vi "Trim end of multiline string of CRLFs and just have one CRLF.vi"(8 "error in (no error)":errorcluster, 11 "String in":string) -> (0 "error out":errorcluster, 1 "Delimiter":string, 2 "String out":string, 3 "Line cnt":i32)   [LabVIEW 2013]
doc: "Removes end of multiline string whitespace on just the last line and puts one lf there so string is just the number of lines it should be, returns count of lines too. This is intended for processing csv line recs file. Also determine the delimiter character between fields. This does some processing of an entire text string which is the read of all file chars. Lines will be processed with pick line vi and loop index."
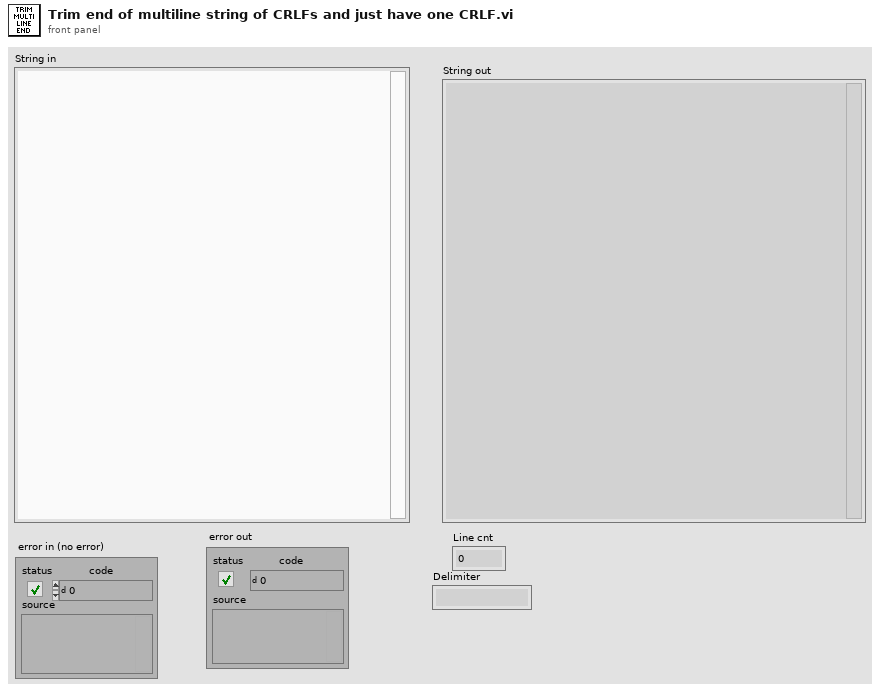
[diagram p1: front panel]
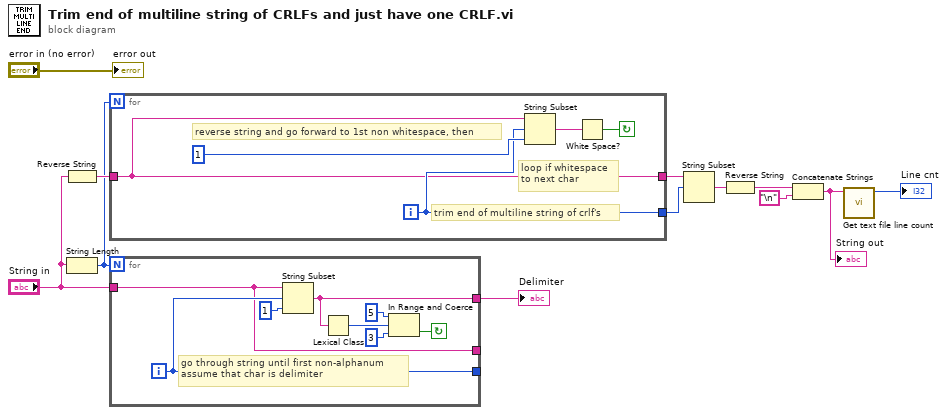
[diagram p0: block diagram]
diagram:
  n1 = Reverse String(1:"String in") -> (0:w9:string)
  n2 = String Length(string="String in") -> (length=w2:i32)
  n3 = for {
    N: w2 -> [_]
    tunnel: w9 -> [w13]
    tunnel: [w14] -> w8
    tunnel: [w13] -> w12
    i -> [w14]
    stop <- w15 continue-if-true
    # "loop if whitespace\nto next char"
    # "reverse string and go forward to 1st non whitespace, then"
    # "trim end of multiline string of crlf's"
    n4 = String Subset(string=w13, offset (0)=w14, length (rest)=1 ("length (rest)")) -> (substring=w16:string)
    n5 = White Space?(1:w16) -> (0:w15:bool)
  }
  n6 = for {
    N: w2 -> [_]
    tunnel: "String in" -> [w23]
    tunnel: [w24] -> _
    tunnel: [w23] -> _
    tunnel: [w18] -> w1
    i -> [w24]
    stop <- w19 continue-if-true
    # "go through string until first non-alphanum\nassume that char is delimiter"
    n7 = String Subset(string=w23, offset (0)=w24, length (rest)=1 ("length (rest)")) -> (substring=w18:string)
    n8 = Lexical Class(1:w18) -> (0:w22:i16)
    n9 = In Range and Coerce(upper limit=i16 5, x=w22, lower limit=i16 3) -> (In Range?=w19:bool)  [unwired: 1 out]
  }
  "Delimiter" <- w1
  n10 = String Subset(string=w12, offset (0)=w8) -> (substring=w10:string)  [unwired: 1 in]
  n11 = Reverse String(1:w10) -> (0:w11:string)
  n12 = Concatenate Strings(w11, "\n") -> (w7:string)
  "String out" <- w7
  n13 = call "Get text file line count.vi"("text string"=w7) -> ("Line cnt"=→"Line cnt":i32)  [unwired: 9 in, 1 out]
  "error out" <- "error in (no error)"
